vi "Read Data.vi"(7 "初始化?":bool, 8 "error in (no error)":errorcluster caption="错误输入（无错误）", 11 "虚拟 输入":refnum<class "虚拟.lvclass">) -> (0 "error out":errorcluster caption="错误输出", 1 "完成":bool, 2 "DBL":dbl[][](array[numeric]), 3 "虚拟 输出":refnum<class "虚拟.lvclass">)   [LabVIEW 2020, in "虚拟.lvclass"]
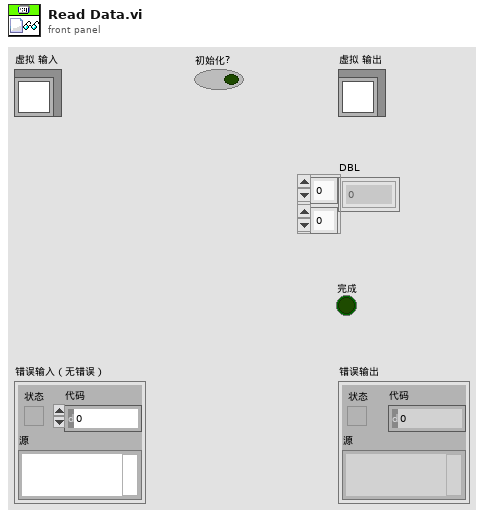
[diagram p1: front panel]
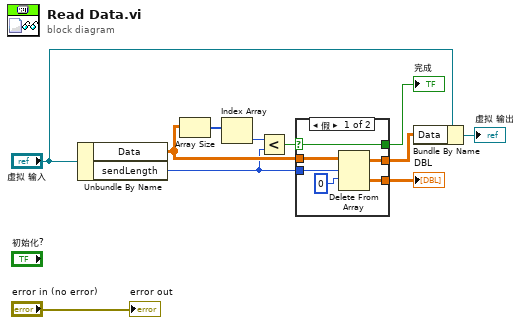
[diagram p0: block diagram]
diagram:
  n1 = Unbundle By Name("虚拟 输入") -> ("Data"=w6:dbl[][], "sendLength"=w3:i32)
  n2 = Array Size(array=w6) -> (size(s)=w5:i32[])
  n3 = Index Array(array=w5) -> (element=w4:i32)  [unwired: 1 in]
  n4 = Less?(x=w4, y=w3) -> (x < y?=w2:bool)
  n5 = case shown="假" w2 {
    selector: w2 -> [w12 w18]
    tunnel: w6 -> [w17 w19]
    tunnel: w3 -> [w16 _]
    tunnel: [w14 _] -> w8
    tunnel: [w13 w19] -> w7
    tunnel: [w12 w18] -> w1
    frame False {
      n6 = Delete From Array(array=w17, length=w16, index (row)=0 ("索引 (行)")) -> (deleted portion=w13:dbl[][], array with subset deleted=w14:dbl[][])  [unwired: 1 in]
    }
    frame True {
    }
  }
  "DBL" <- w7
  "完成" <- w1
  n7 = Bundle By Name(cluster="虚拟 输入", "Data"=w8) -> (→"虚拟 输出":refnum<class "虚拟.lvclass">)
  "error out" <- "error in (no error)"
